vi "mono-shutter.vi"(8 "error in (no error)":errorcluster, 10 "Set":bool, 11 "Monochromator":refnum<vi>) -> (0 "error out":errorcluster)   [LabVIEW 2016]
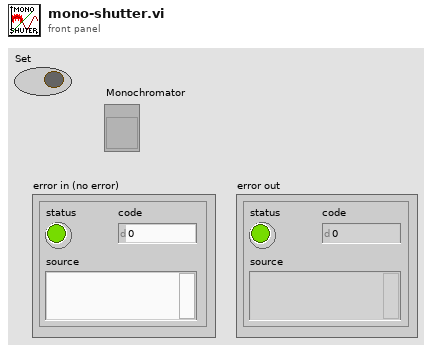
[diagram p1: front panel]
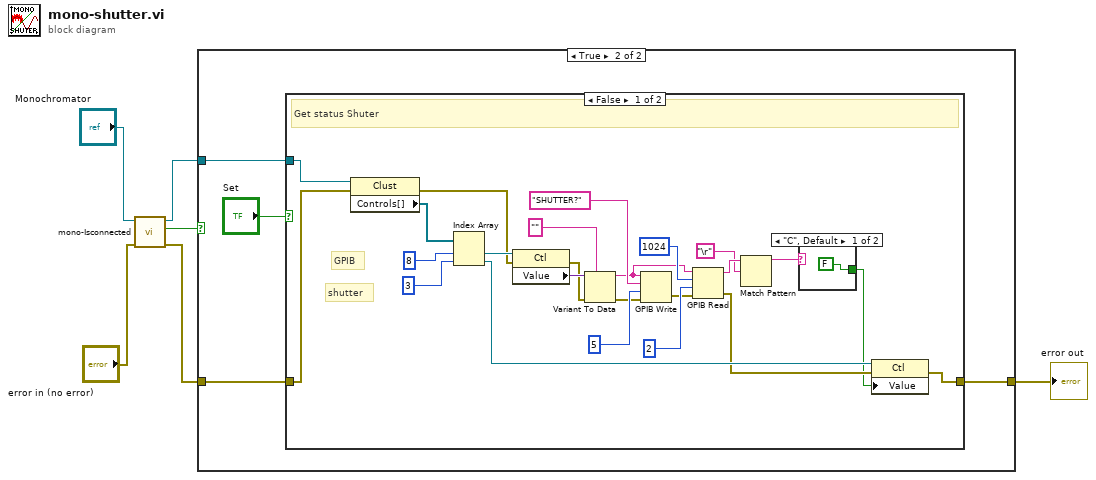
[diagram p0: block diagram]
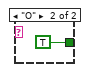
[diagram p3: hidden frame]
diagram:
  n1 = call "mono-Isconnected.vi"("error in (no error)"="error in (no error)", "Monochromator"="Monochromator") -> ("error out"=w6:errorcluster, "Connected"=w2:bool, "Monochromator out"=w3:refnum<vi>)  [unwired: 7 in]
  n2 = case shown="True" w2 {
    tunnel: w6 -> [w7 w8]
    tunnel: w3 -> [_ w10]
    tunnel: [w7 w9] -> w1
    frame False {
    }
    frame True {
      n3 = case shown="False" "Set" {
        tunnel: w10 -> [w35 _]
        tunnel: [w13 w38] -> w9
        tunnel: w8 -> [w12 w38]
        frame False {
          # "shutter"
          # "GPIB"
          # "Get status Shuter"
          n4 = property class="Clust"(reference=w35, error in=w12) -> (error out=w31:errorcluster, "Controls[]"=w34:refnum<vi>[])  [unwired: 1 out]
          n5 = Index Array(array=w34, index #1=8 ("index"), index #2=3 ("index")) -> (element #1=w32:refnum<vi>, element #2=w16:refnum<vi>)
          n6 = property class="Ctl"(reference=w32, error in=w31) -> (error out=w29:errorcluster, "Value"=w30:variant)  [unwired: 1 out]
          n7 = Variant To Data(error in=w29, type="", Variant=w30) -> (data=w19:string, error out=w20:errorcluster)
          n8 = GPIB Write(0:w19, 1:"SHUTTER?" ("data"), 2:i16 5 ("mode (0)"), 3:w20) -> (6:w25:errorcluster)  [unwired: 1 in, 1 out]
          n9 = GPIB Read(0:w19, 1:1024 ("byte count"), 2:i16 2 ("mode (0)"), 3:w25) -> (5:w22:string, 7:w15:errorcluster)  [unwired: 1 in, 1 out]
          n10 = Match Pattern(string=w22, regular expression="\r") -> (before substring=w18:string)  [unwired: 1 in, 3 out]
          n11 = case shown="\"C\", Default" w18 {
            tunnel: [FALSE TRUE] -> w14
            frame "C", Default {
            }
            frame "O" {
            }
          }
          n12 = property class="Ctl"(reference=w16, error in=w15, "Value"=w14) -> (error out=w13:errorcluster)  [unwired: 1 out]
        }
        frame True {
          # "Set status Shutter"
        }
      }
    }
  }
  "error out" <- w1
